vi "writetofile.vi"(6 "FilePath":refnum<vi>, 7 "Save Flag Reference":refnum<vi>, 8 "error in (no error)":errorcluster, 9 "Rec Flag Reference":refnum<vi>, 10 "Stop Flag Reference":refnum<vi>, 11 "QuadraturePositionDecoder in":refnum<class "QuadraturePositionDecoder.lvclass">) -> (0 "error out":errorcluster, 3 "QuadraturePositionDecoder out":refnum<class "QuadraturePositionDecoder.lvclass">)   [LabVIEW 2014, in "QuadraturePositionDecoder.lvclass"]
uses:
  QuadraturePositionDecoder.lvclass
  QuadraturePositionDecoder.lvclass/QuadraturePositionDecoder.ctl
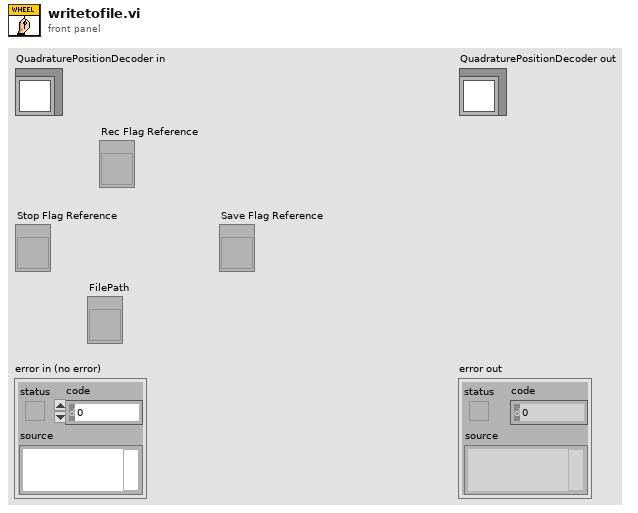
[diagram p1: front panel]
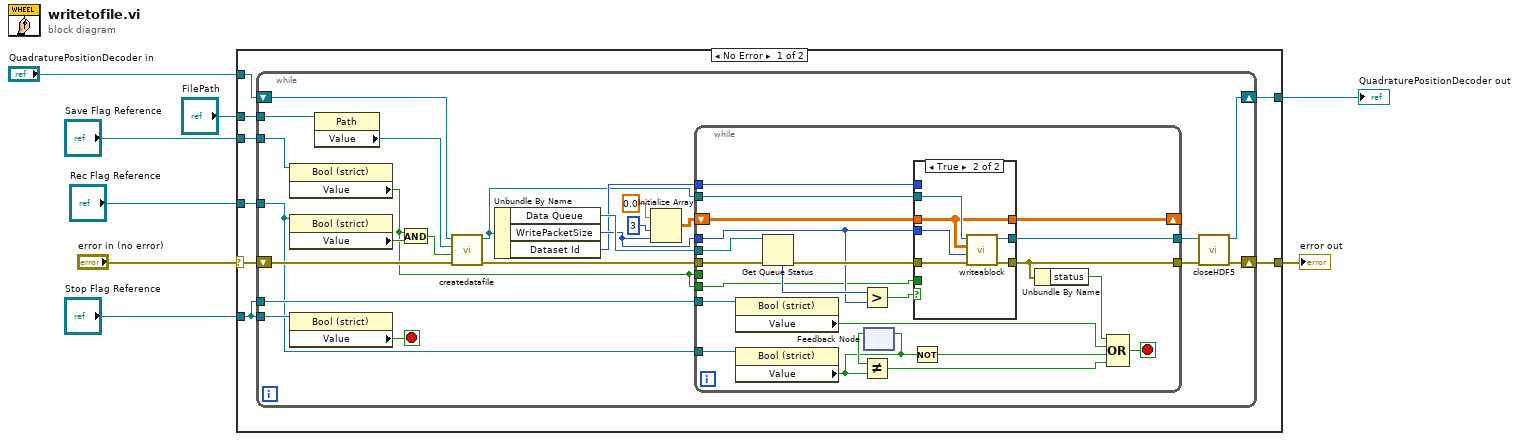
[diagram p0: block diagram]
diagram:
  n1 = case shown="No Error" "error in (no error)" {
    selector: "error in (no error)" -> [w16 w73]
    tunnel: [w15 w73] -> w7
    tunnel: [w13 w72] -> w5
    tunnel: "QuadraturePositionDecoder in" -> [w14 w72]
    tunnel: "Stop Flag Reference" -> [w12 _]
    tunnel: "Rec Flag Reference" -> [w11 _]
    tunnel: "FilePath" -> [w10 _]
    tunnel: "Save Flag Reference" -> [w9 _]
    frame No Error {
      n2 = while {
        tunnel: w12 -> [w40]
        shift-right: [w22] -> w15
        shift-left: w16 -> [w31]
        shift-right: [w23] -> w13
        shift-left: w14 -> [w33]
        tunnel: w12 -> [w29]
        tunnel: w11 -> [w28]
        tunnel: w10 -> [w27]
        tunnel: w9 -> [w17]
        stop <- w19 stop-if-true
        n3 = property class="Bool (strict)"(reference=w17) -> ("Value"=w18:bool)  [unwired: 1 in, 2 out]
        n4 = property class="Bool (strict)"(reference=w28) -> ("Value"=w21:bool)  [unwired: 1 in, 2 out]
        n5 = property class="Bool (strict)"(reference=w29) -> ("Value"=w19:bool)  [unwired: 1 in, 2 out]
        n6 = property class="Path"(reference=w27) -> ("Value"=w26:path)  [unwired: 1 in, 2 out]
        n7 = And(x=w18, y=w21) -> (x .and. y?=w20:bool)
        n8 = call-dynamic "createdatafile.vi"("error in (no error)"=w31, "Save Wheel"=w20, "path"=w26, "QuadraturePositionDecoder in"=w33) -> ("error out"=w30:errorcluster, "QuadraturePositionDecoder out"=w32:refnum<class "QuadraturePositionDecoder.lvclass">)  [unwired: 6 in]
        n9 = Unbundle By Name(w32) -> ("Data Queue"=w38:refnum<queue>, "WritePacketSize"=w35:i32, "Dataset Id"=w34:i32)
        n10 = Initialize Array(0.0 ("element"), 3 ("dimension size"), w35) -> (w36:dbl[][])
        n11 = while {
          tunnel: w30 -> [w62]
          tunnel: [w59] -> w25
          tunnel: w40 -> [w60]
          tunnel: w38 -> [w56]
          tunnel: w35 -> [w54]
          shift-right: [w51] -> _
          shift-left: w36 -> [w55]
          tunnel: w18 -> [w53]
          tunnel: w34 -> [w52]
          tunnel: w32 -> [w50]
          tunnel: [w49] -> w24
          tunnel: w28 -> [w45]
          tunnel: w18 -> [_]
          stop <- w46 stop-if-true
          n12 = property class="Bool (strict)"(reference=w60) -> ("Value"=w47:bool)  [unwired: 1 in, 2 out]
          n13 = property class="Bool (strict)"(reference=w45) -> ("Value"=w42:bool)  [unwired: 1 in, 2 out]
          n14 = Get Queue Status(queue=w56, error in (no error)=w62) -> (error out=w61:errorcluster, # elements in queue=w58:i32)  [unwired: 1 in, 6 out]
          n15 = Greater?(x=w58, y=w54) -> (0:w57:bool)
          n16 = feedback #1() -> (w43:bool)  [unwired: 1 in]
          n17 = Not Equal?(x=w43, y=w42) -> (x != y?=w41:bool)
          n18 = feedback-in #1(w42) -> ()
          n19 = Not(x=w42) -> (.not. x?=w44:bool)
          n20 = case shown="True" w57 {
            tunnel: w61 -> [w65 w68]
            tunnel: [w65 w67] -> w59
            tunnel: w54 -> [_ w69]
            tunnel: w55 -> [w64 w66]
            tunnel: w53 -> [_ _]
            tunnel: w52 -> [_ _]
            tunnel: [w64 w66] -> w51
            tunnel: w50 -> [w63 w71]
            tunnel: [w63 w70] -> w49
            frame False {
            }
            frame True {
              n21 = call-dynamic "writeablock.vi"("error in (no error)"=w68, "BlockSize"=w69, "Array"=w66, "QuadraturePositionDecoder in"=w71) -> ("error out"=w67:errorcluster, "QuadraturePositionDecoder out"=w70:refnum<class "QuadraturePositionDecoder.lvclass">)  [unwired: 6 in]
            }
          }
          n22 = Unbundle By Name(w59) -> ("status"=w48:bool)
          n23 = Compound Arithmetic op=OR(w48, w47, w44, w41) -> (w46:bool)
        }
        n24 = call-dynamic "closeHDF5.vi"("error in (no error)"=w25, "QuadraturePositionDecoder in"=w24) -> ("error out"=w22:errorcluster, "QuadraturePositionDecoder out"=w23:refnum<class "QuadraturePositionDecoder.lvclass">)  [unwired: 8 in]
      }
    }
    frame Error {
    }
  }
  "error out" <- w7
  "QuadraturePositionDecoder out" <- w5
